vi "Color to Color Hex.vi"(11 "Color":u32(colorbox)) -> (3 "Hex Color":string)   [LabVIEW 2023, in "Confluence Formatting.lvlib"]
uses:
  Confluence Formatting.lvlib
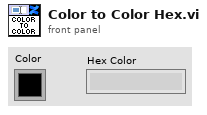
[diagram p1: front panel]
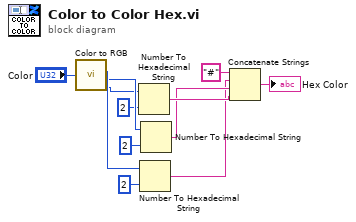
[diagram p0: block diagram]
diagram:
  n1 = call <vilib>:"Color to RGB.vi"("Color"="Color") -> ("R"=w6:u8, "G"=w5:u8, "B"=w1:u8)  [unwired: 1 out]
  n2 = Number To Hexadecimal String(1:i16 2 ("width (-)"), 2:w1) -> (0:w9:string)
  n3 = Number To Hexadecimal String(1:i16 2 ("width (-)"), 2:w6) -> (0:w7:string)
  n4 = Number To Hexadecimal String(1:i16 2 ("width (-)"), 2:w5) -> (0:w8:string)
  n5 = Concatenate Strings("#" ("string"), w7, w8, w9) -> (→"Hex Color":string)
